vi "Intake Shooter Immediate.vi"(7 "Description":string, 8 "Command Info In":T1, 11 "Intake joystick":dbl) -> (0 "Command Info Out":T1)   [LabVIEW 2019]
doc: "This template is useful for immediate subsystem actions that do not need deadband filtering\n\nBe sure to right-click and select New from Template and save with a new command name."
uses:
  <vilib>/Rock Robotics/WPI/Framework/Command Status Info.ctl
  <vilib>/Rock Robotics/WPI/Framework/Completion Status.ctl
  <vilib>/Rock Robotics/WPI/Framework/Completion Notifier.ctl
  Implementation/Intake Shooter Operations.ctl
  Implementation/Intake Shooter Setpoints.ctl
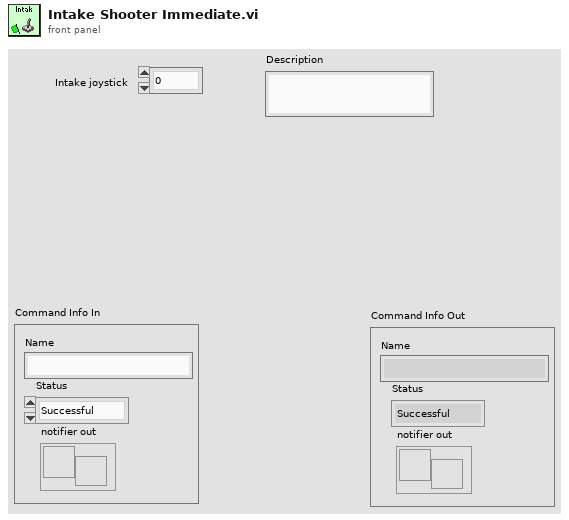
[diagram p1: front panel]
types:
  T1 = typedef "Command Status Info.ctl" = cluster{"Name":string, "Status":T2, "notifier out":T3}
  T2 = typedef "Completion Status.ctl" = enum16{"Successful", "Aborted", "Incomplete"}
  T3 = typedef "Completion Notifier.ctl" = refnum<notifier>
  T4 = typedef "Intake Shooter Operations.ctl" = enum16{"Reserve", "Read Current", "Immediate", "Go up", "Go down", "Armediate"}
  T5 = typedef "Intake Shooter Setpoints.ctl" = cluster{"Operation":T4, "Intake setpoint":dbl, "Duration":dbl, "Tilt setpoint":dbl, "Speed":dbl, "Distance":dbl}
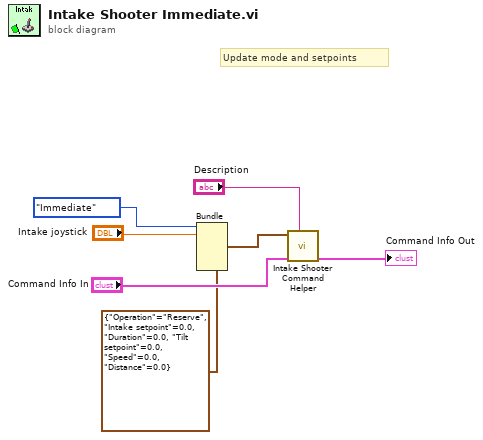
[diagram p0: block diagram]
diagram:
  # "Update mode and setpoints"
  n1 = Bundle(cluster=T5 {"Operation"=enum."Reserve", "Intake setpoint"=0.0, "Duration"=0.0, "Tilt setpoint"=0.0, "Speed"=0.0, "Distance"=0.0} ("SubSystem Data"), "Operation"=Intake_Shooter_Operations."Immediate", "Intake setpoint"="Intake joystick") -> (w2:T5)  [unwired: 4 in]
  n2 = call "Intake Shooter Command Helper.vi"("Description"="Description", "Command Info In"="Command Info In", "SubSystem Data"=w2) -> ("Command Info Out"=→"Command Info Out":T1)  [unwired: 6 in, 2 out]
